vi "Z Value to Color.vi"(1 "Scale":T1=enum."RWB", 2 "Numeric":dbl) -> (6 "Color":u32)   [LabVIEW 2009]
doc: "This VI converts a single value between 0 and 255 to a color based upon a specified scale."
uses:
  Controls/Color Scales.ctl
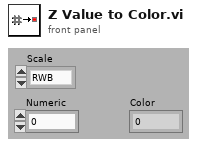
[diagram p1: front panel]
types:
  T1 = typedef "Color Scales.ctl" = enum16{"RGB", "RWB", "BGR", "BWR", "BW", "WB"}
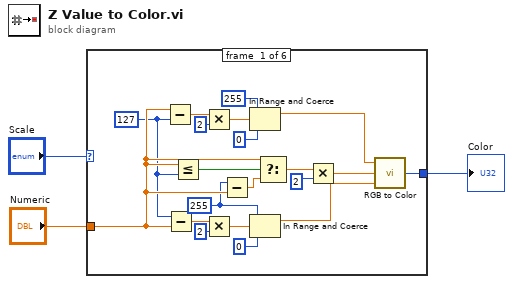
[diagram p0: block diagram]
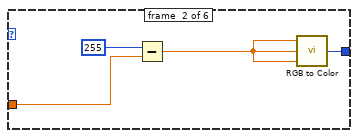
[diagram p2: hidden frame]
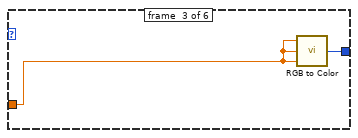
[diagram p3: hidden frame]
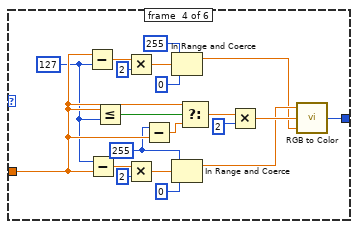
[diagram p4: hidden frame]
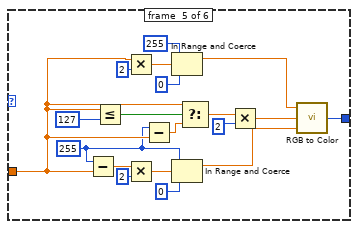
[diagram p5: hidden frame]
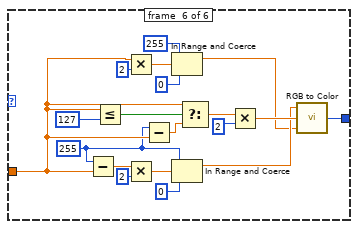
[diagram p6: hidden frame]
diagram:
  n1 = case shown="\"BGR\"" "Scale" {
    tunnel: [w23 w27 w29 w49 w68 w87] -> w3
    tunnel: "Numeric" -> [w22 w25 w28 w48 w51 w72]
    frame #0 {
      w15 = 255 ("upper limit")
      w21 = 127 ("y")
      n2 = Subtract(x=w22, y=w21) -> (x-y=w12:dbl)
      n3 = Subtract(x=w21, y=w22) -> (x-y=w13:dbl)
      n4 = Less Or Equal?(x=w22, y=w21) -> (x <= y?=w11:bool)
      n5 = Multiply(x=w12, y=2) -> (x*y=w6:dbl)
      n6 = Multiply(x=w13, y=2) -> (x*y=w14:dbl)
      n7 = Subtract(x=w15, y=w22) -> (x-y=w16:dbl)
      n8 = In Range and Coerce(upper limit=255, x=w6, lower limit=0) -> (coerced(x)=w10:dbl)  [unwired: 1 out]
      n9 = In Range and Coerce(upper limit=w15, x=w14, lower limit=0) -> (coerced(x)=w17:dbl)  [unwired: 1 out]
      n10 = Select(t=w22, s=w11, f=w16) -> (s? t:f=w18:dbl)
      n11 = Multiply(x=w18, y=2) -> (x*y=w19:dbl)
      n12 = call <vilib>:"RGB to Color.vi"("B"=w17, "G"=w19, "R"=w10) -> ("Color"=w23:u32)
    }
    frame #1 {
      n13 = Subtract(x=255, y=w25) -> (x-y=w24:dbl)
      n14 = call <vilib>:"RGB to Color.vi"("B"=w24, "G"=w24, "R"=w24) -> ("Color"=w27:u32)
    }
    frame #2 {
      n15 = call <vilib>:"RGB to Color.vi"("B"=w28, "G"=w28, "R"=w28) -> ("Color"=w29:u32)
    }
    frame #3 {
      w42 = 255 ("upper limit")
      w47 = 127 ("y")
      n16 = Subtract(x=w48, y=w47) -> (x-y=w39:dbl)
      n17 = Subtract(x=w47, y=w48) -> (x-y=w40:dbl)
      n18 = Less Or Equal?(x=w48, y=w47) -> (x <= y?=w38:bool)
      n19 = Multiply(x=w39, y=2) -> (x*y=w34:dbl)
      n20 = Multiply(x=w40, y=2) -> (x*y=w41:dbl)
      n21 = Subtract(x=w42, y=w48) -> (x-y=w43:dbl)
      n22 = In Range and Coerce(upper limit=255, x=w34, lower limit=0) -> (coerced(x)=w30:dbl)  [unwired: 1 out]
      n23 = In Range and Coerce(upper limit=w42, x=w41, lower limit=0) -> (coerced(x)=w31:dbl)  [unwired: 1 out]
      n24 = Select(t=w48, s=w38, f=w43) -> (s? t:f=w44:dbl)
      n25 = Multiply(x=w44, y=2) -> (x*y=w45:dbl)
      n26 = call <vilib>:"RGB to Color.vi"("B"=w30, "G"=w45, "R"=w31) -> ("Color"=w49:u32)
    }
    frame #4 {
      w50 = 255 ("upper limit")
      n27 = Subtract(x=w50, y=w51) -> (x-y=w60:dbl)
      n28 = Less Or Equal?(x=w51, y=127) -> (x <= y?=w59:bool)
      n29 = Multiply(x=w51, y=2) -> (x*y=w54:dbl)
      n30 = Multiply(x=w60, y=2) -> (x*y=w61:dbl)
      n31 = Subtract(x=w50, y=w51) -> (x-y=w62:dbl)
      n32 = In Range and Coerce(upper limit=255, x=w54, lower limit=0) -> (coerced(x)=w58:dbl)  [unwired: 1 out]
      n33 = In Range and Coerce(upper limit=w50, x=w61, lower limit=0) -> (coerced(x)=w63:dbl)  [unwired: 1 out]
      n34 = Select(t=w51, s=w59, f=w62) -> (s? t:f=w64:dbl)
      n35 = Multiply(x=w64, y=2) -> (x*y=w65:dbl)
      n36 = call <vilib>:"RGB to Color.vi"("B"=w63, "G"=w65, "R"=w58) -> ("Color"=w68:u32)
    }
    frame #5 {
      w71 = 255 ("upper limit")
      n37 = Subtract(x=w71, y=w72) -> (x-y=w80:dbl)
      n38 = Less Or Equal?(x=w72, y=127) -> (x <= y?=w79:bool)
      n39 = Multiply(x=w72, y=2) -> (x*y=w75:dbl)
      n40 = Multiply(x=w80, y=2) -> (x*y=w81:dbl)
      n41 = Subtract(x=w71, y=w72) -> (x-y=w82:dbl)
      n42 = In Range and Coerce(upper limit=255, x=w75, lower limit=0) -> (coerced(x)=w69:dbl)  [unwired: 1 out]
      n43 = In Range and Coerce(upper limit=w71, x=w81, lower limit=0) -> (coerced(x)=w70:dbl)  [unwired: 1 out]
      n44 = Select(t=w72, s=w79, f=w82) -> (s? t:f=w83:dbl)
      n45 = Multiply(x=w83, y=2) -> (x*y=w84:dbl)
      n46 = call <vilib>:"RGB to Color.vi"("B"=w69, "G"=w84, "R"=w70) -> ("Color"=w87:u32)
    }
  }
  "Color" <- w3
